vi "MGCC_FntStaMach_main.vi"() -> ()   [LabVIEW 2016]
doc: "Main function for FSM in MGCC. The inputs are flags feedback from other functions and MGLCs. The outputs are the next states and updates in sensoring datas."
panel:
  in  "b_MGCC_FntStaMach_All_Loop_Stop":bool
  out "Functions":bool[](array[boolean])
  out "Current state":string
  out "Current Time":string
  in  "Manual turn off":bool
  in  "Event manual panel":bool
  out "Bool of state":bool[](array[boolean])
  # "Finte State Machine"
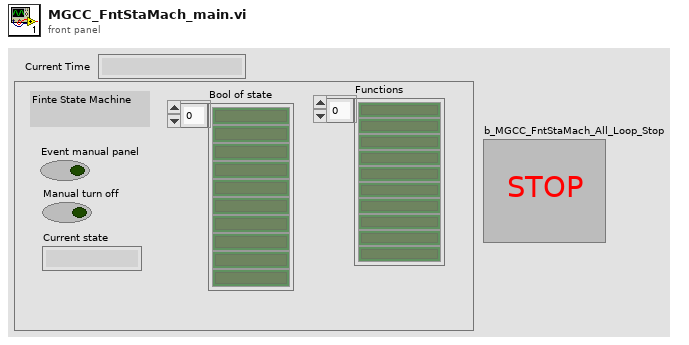
[diagram p1: front panel]
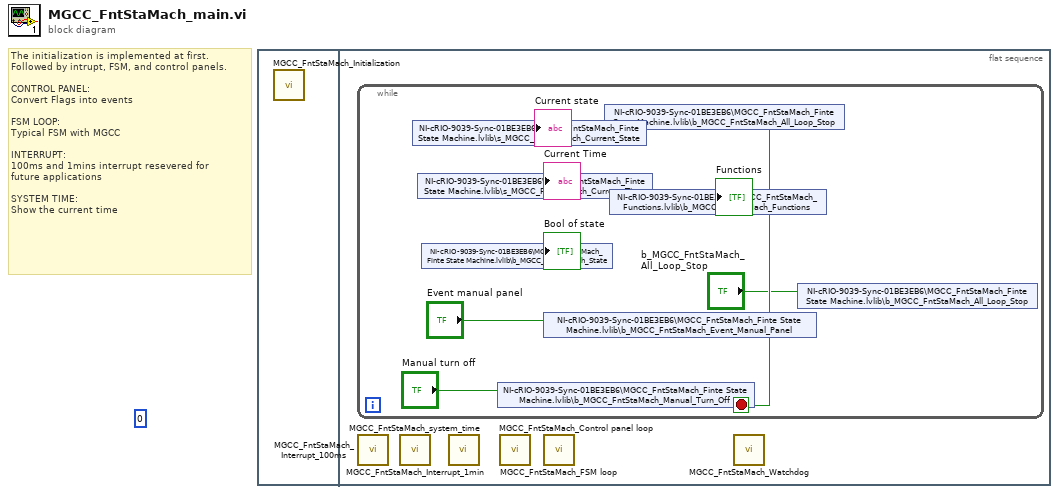
[diagram p0: block diagram]
diagram:
  (unwired) 0
  # "The initialization is implemented at first.\nFollowed by intrupt, FSM, and control panels.\n\nCONTROL PANEL:\nConvert Flags into events\n\nFSM LOOP:\nTypical FSM with MGCC\n\nINTERRUPT:\n100ms and 1mins interrupt resevered for \nfuture applications\n\nSYSTEM TIME:\nShow the current time"
  n1 = flat-sequence {
    frame #0 {
      n2 = call "MGCC_FntStaMach_Initialization.vi"() -> ()  [unwired: 12 in]
    }
    frame #1 {
      n3 = while {
        stop <- w7 stop-if-true
        n4 = shared-variable "NI-cRIO-9039-Sync-01BE3EB6\\MGCC_FntStaMach_Finte State Machine.lvlib\\s_MGCC_FntStaMach_Current_State"() -> (→"Current state":string)  [unwired: 1 in, 1 out]
        n5 = shared-variable "NI-cRIO-9039-Sync-01BE3EB6\\MGCC_FntStaMach_Finte State Machine.lvlib\\s_MGCC_FntStaMach_Current_Time"() -> (→"Current Time":string)  [unwired: 1 in, 1 out]
        n6 = shared-variable "NI-cRIO-9039-Sync-01BE3EB6\\MGCC_FntStaMach_Finte State Machine.lvlib\\b_MGCC_FntStaMach_State"() -> (→"Bool of state":bool[])  [unwired: 1 in, 1 out]
        n7 = shared-variable "NI-cRIO-9039-Sync-01BE3EB6\\MGCC_FntStaMach_Finte State Machine.lvlib\\b_MGCC_FntStaMach_Manual_Turn_Off"("Manual turn off") -> ()  [unwired: 1 in, 1 out]
        n8 = shared-variable "NI-cRIO-9039-Sync-01BE3EB6\\MGCC_FntStaMach_Finte State Machine.lvlib\\b_MGCC_FntStaMach_Event_Manual_Panel"("Event manual panel") -> ()  [unwired: 1 in, 1 out]
        n9 = shared-variable "NI-cRIO-9039-Sync-01BE3EB6\\MGCC_FntStaMach_Finte State Machine.lvlib\\b_MGCC_FntStaMach_All_Loop_Stop"() -> (w7:bool)  [unwired: 1 in, 1 out]
        n10 = shared-variable "NI-cRIO-9039-Sync-01BE3EB6\\MGCC_FntStaMach_Functions.lvlib\\b_MGCC_FntStaMach_Functions"() -> (→"Functions":bool[])  [unwired: 1 in, 1 out]
        n11 = shared-variable "NI-cRIO-9039-Sync-01BE3EB6\\MGCC_FntStaMach_Finte State Machine.lvlib\\b_MGCC_FntStaMach_All_Loop_Stop"("b_MGCC_FntStaMach_All_Loop_Stop") -> ()  [unwired: 1 in, 1 out]
      }
      n12 = call "MGCC_FntStaMach_Interrupt_100ms.vi"() -> ()  [unwired: 11 in, 1 out]
      n13 = call "MGCC_FntStaMach_Interrupt_1min.vi"() -> ()  [unwired: 11 in, 1 out]
      n14 = call "MGCC_FntStaMach_system_time.vi"() -> ()  [unwired: 12 in]
      n15 = call "MGCC_FntStaMach_Control panel loop.vi"() -> ()  [unwired: 12 in]
      n16 = call "MGCC_FntStaMach_FSM loop.vi"() -> ()  [unwired: 6 in, 6 out]
      n17 = call "MGCC_FntStaMach_Watchdog.vi"() -> ()  [unwired: 12 in]
    }
  }
